vi "Writer.vi"(9 "Color Settings":T1, 10 "FileName":string="Blue2.csv", 11 "FilePath":path=path "C:/Program Files (x86)/FRC Dashboard") -> ()   [LabVIEW 2013]
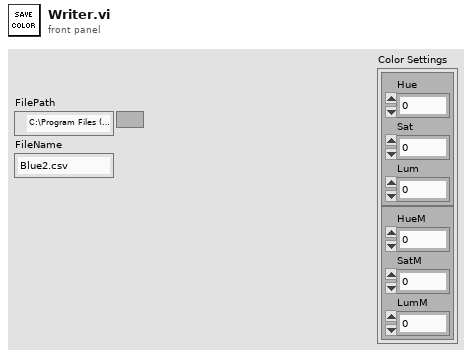
[diagram p1: front panel]
types:
  T1 = cluster{cluster{"Hue":i32, "Sat":i32, "Lum":i32}, cluster{"HueM":i32, "SatM":i32, "LumM":i32}}
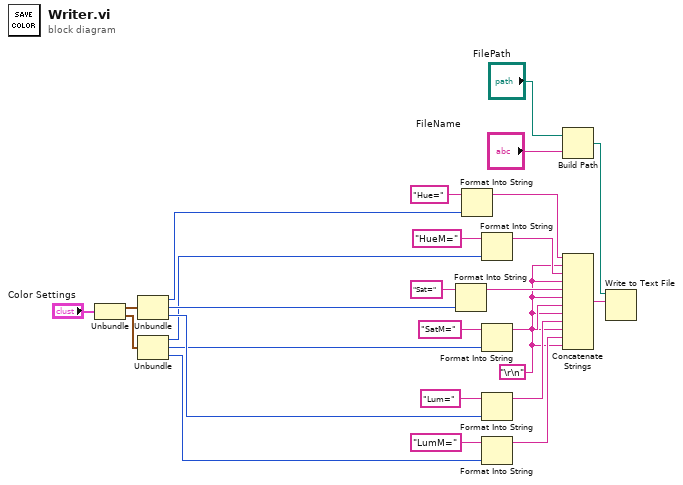
[diagram p0: block diagram]
diagram:
  w12 = "\r\n"
  n1 = Unbundle("Color Settings") -> (w7:cluster{"Hue":i32, "Sat":i32, "Lum":i32}, w8:cluster{"HueM":i32, "SatM":i32, "LumM":i32})
  n2 = Unbundle(w7) -> ("Hue"=w6:i32, "Sat"=w5:i32, "Lum"=w4:i32)
  n3 = Unbundle(w8) -> ("HueM"=w3:i32, "SatM"=w2:i32, "LumM"=w1:i32)
  n4 = Format Into String(initial string="Sat=", w5) -> (resulting string=w15:string)  [unwired: 2 in, 1 out]
  n5 = Format Into String(initial string="Hue=", w6) -> (resulting string=w25:string)  [unwired: 2 in, 1 out]
  n6 = Format Into String(initial string="HueM=", w3) -> (resulting string=w23:string)  [unwired: 2 in, 1 out]
  n7 = Format Into String(initial string="SatM=", w2) -> (resulting string=w20:string)  [unwired: 2 in, 1 out]
  n8 = Format Into String(initial string="Lum=", w4) -> (resulting string=w14:string)  [unwired: 2 in, 1 out]
  n9 = Format Into String(initial string="LumM=", w1) -> (resulting string=w13:string)  [unwired: 2 in, 1 out]
  n10 = Build Path(base path="FilePath", name or relative path="FileName") -> (appended path=w10:path)
  n11 = Concatenate Strings(w25, w12, w23, w12, w15, w12, w20, w12, w14, w12, w13, w12) -> (w11:string)
  n12 = Write to Text File(file (use dialog)=w10, text=w11) -> ()  [unwired: 2 in, 3 out]
